vi "HFRR ADV v11.vi"() -> ()   [LabVIEW 2025] (continued)
          frame True {
          }
        }
        n2643 = In Range and Coerce(upper limit=w3178, x=w3151, lower limit=w3177) -> (In Range?=w3169:bool)  [unwired: 1 out]
        n2644 = In Range and Coerce(upper limit=w3175, x=w3150, lower limit=w3176) -> (In Range?=w3167:bool)  [unwired: 1 out]
        n2645 = case shown="True" w3183 {
          frame False {
            n2646 = local read "Rt 3"() -> (w3311:bool)
            n2647 = case shown="True" w3311 {
              frame False {
              }
              frame True {
                n2648 = local write "Rt 3"(FALSE ("Rt 3")) -> ()
                n2649 = local write "Json End Flg"(TRUE ("Upld AR 2")) -> ()
              }
            }
            "Rt" <- TRUE ("Rt")
            "Rt 2" <- FALSE ("Rt")
          }
          frame True {
            n2650 = local read "Rt"() -> (w3318:bool)
            n2651 = local write "Rt 2"(TRUE ("Rt 2")) -> ()
            n2652 = case shown="True" w3318 {
              frame False {
              }
              frame True {
                w3319 = TRUE ("Upld AR 2")
                n2653 = local write "Rt"(FALSE ("Rt")) -> ()
                n2654 = local write "Upld AR"(w3319) -> ()
                n2655 = local write "Json St Flg"(w3319) -> ()
              }
            }
            "Rt 3" <- TRUE ("Rt 3")
          }
        }
        n2656 = case shown="True" w3169 {
          tunnel: [FALSE ("RUN") TRUE ("RUN")] -> w3168
          tunnel: [_ 2] -> w3162
          frame False {
          }
          frame True {
          }
        }
        n2657 = case shown="True" w3167 {
          tunnel: [FALSE ("RUN") TRUE ("RUN")] -> w3166
          tunnel: [_ 3] -> w3161
          frame False {
          }
          frame True {
          }
        }
        n2658 = case shown="\"Acquire\"" w3147 {
          tunnel: w3149 -> [_ w3380]
          frame Default {
            w3379 = 0.0 ("output")
            n2659 = local write "PID-out"(w3379) -> ()
            n2660 = local write "Frequency ( Hz )"(w3379) -> ()
          }
          frame "Acquire" {
            n2661 = stacked-sequence {
              frame #0 {
                n2662 = local read "Auto Start Test"() -> (w3382:bool)
                n2663 = case shown="True" w3382 {
                  tunnel: "RUN" -> [w3403 w3406]
                  tunnel: [w3403 w3405] -> w3383
                  frame False {
                  }
                  frame True {
                    n2664 = local read "Auto Start Temp"() -> (w3404:bool)
                    n2665 = Or(x=w3406, y=w3404) -> (x .or. y?=w3405:bool)
                  }
                }
                n2666 = local read "clk"() -> (w3402:dbl)
                n2667 = local read "Save"() -> (w3398:bool)
                n2668 = Equal?(x=w3402, y=0.0) -> (x = y?=w3399:bool)
                n2669 = And(x=w3399, y=w3398) -> (x .and. y?=w3400:bool)
                n2670 = Not(x="Engage") -> (.not. x?=w3389:bool)
                n2671 = case shown="True" w3383 {
                  tunnel: [w3414 w3432] -> w3385
                  frame False {
                    w3414 = 0.0
                    n2672 = local read "Auto Start Test"() -> (w3410:bool)
                    n2673 = local write "Reinit PID"(TRUE) -> ()
                    n2674 = local write "Start Time"(TRUE ("Start Time")) -> ()
                    n2675 = property on="Stroke" class="DigNum (strict)"("Visible"=TRUE) -> ()  [unwired: 2 in, 2 out]
                    n2676 = property on="Stroke 2" class="DigNum (strict)"("Visible"=FALSE) -> ()  [unwired: 2 in, 2 out]
                    n2677 = case shown="False" w3410 {
                      frame False {
                        n2678 = property on="Heater Button" class="Bool (strict)"("DisabledEnum"=T16."Enabled" ("Disabled")) -> ()  [unwired: 2 in, 2 out]
                        n2679 = property on="Humidity" class="Bool (strict)"("DisabledEnum"=T16."Enabled" ("Disabled")) -> ()  [unwired: 2 in, 2 out]
                      }
                      frame True {
                      }
                    }
                    n2680 = case shown="False" "TestCompFlg" {
                      frame False {
                        n2681 = local read "StartFlg"() -> (w3420:bool)
                        n2682 = case shown="True" w3420 {
                          frame False {
                          }
                          frame True {
                            n2683 = flat-sequence {
                              frame #0 {
                                n2684 = local read "EVENT LOG"() -> (w3422:string)
                                n2685 = call "Event Log.vi"("Content"="Test was interrupted", "EVENT LOG"=w3422) -> ("EVENT LOG"=w3423:string)  [unwired: 8 in, 1 out]
                                n2686 = local write "EVENT LOG"(w3423) -> ()
                              }
                              frame #1 {
                                w3424 = FALSE ("StartFlg")
                                n2687 = local write "Heater Button"(w3424) -> ()
                                n2688 = local write "StartFlg"(w3424) -> ()
                                n2689 = local write "Humidity"(w3424) -> ()
                              }
                            }
                          }
                        }
                      }
                      frame True {
                      }
                    }
                    n2690 = local write "String 14"("Test will autostart once parameters reach the set value." ("String 14")) -> ()
                    n2691 = local write "Old Pid Val"(w3414) -> ()
                  }
                  frame True {
                    n2692 = property on="Stroke 2" class="DigNum (strict)"("Visible"=TRUE) -> ()  [unwired: 2 in, 2 out]
                    n2693 = property on="Stroke" class="DigNum (strict)"("Visible"=FALSE) -> ()  [unwired: 2 in, 2 out]
                    n2694 = property on="STOP 2" class="Bool (strict)"("Disabled"=u8 2) -> ()  [unwired: 2 in, 2 out]
                    n2695 = local write "String 14"(" Running....." ("String 14")) -> ()
                    n2696 = property on="Heater Button" class="Bool (strict)"("DisabledEnum"=T16."Disabled and Grayed Out" ("Disabled")) -> ()  [unwired: 2 in, 2 out]
                    n2697 = property on="Humidity" class="Bool (strict)"("DisabledEnum"=T16."Disabled and Grayed Out" ("Disabled")) -> ()  [unwired: 2 in, 2 out]
                    n2698 = local read "PID Ref"() -> (w3443:bool)
                    n2699 = case shown="True" w3443 {
                      tunnel: [w3449 w3465] -> w3442
                      frame False {
                        n2700 = local read "Old Pid Val"() -> (w3449:dbl)
                      }
                      frame True {
                        n2701 = local read "Set Hz"() -> (w3458:dbl)
                        n2702 = local read "Frequency"() -> (w3469:dbl)
                        n2703 = Add(x=w3458, y=10.0) -> (x+y=w3467:dbl)
                        n2704 = Add(x=w3458, y=-10.0 ("Offset")) -> (x+y=w3476:dbl)
                        n2705 = Add(x=w3458, y=-10.0) -> (x+y=w3468:dbl)
                        n2706 = In Range and Coerce(upper limit=w3467, x=w3469, lower limit=w3468) -> (coerced(x)=w3457:dbl)  [unwired: 1 out]
                        n2707 = Or(x="Reinit PID", y="Reinit PID") -> (x .or. y?=w3466:bool)
                        n2708 = Multiply(x=w3476, y=0.1 ("Gain")) -> (x*y=w3455:dbl)
                        n2709 = local read "Elapsed time"() -> (w3462:dbl)
                        n2710 = local read "SPEED OUT:"() -> (w3477:dbl)
                        n2711 = Add(x=w3455, y=1.5) -> (x+y=w3453:dbl)
                        n2712 = call-poly <vilib>:"PID.vi"("reinitialize? (F)"=w3466, "output range"=cluster{"output high":dbl, "output low":dbl} {"output high"=1.0, "output low"=-1.0}, "PID gains"=T13 {"proportional gain (Kc)"=0.0005, "integral time (Ti, min)"=0.001, "derivative time (Td, min)"=0.0} ("Motor PID"), "process variable"=w3457, "setpoint"=w3458) -> ("output"=w3456:dbl)  [unwired: 5 in, 1 out]
                        n2713 = Multiply(x=w3453, y=w3477) -> (x*y=w3452:dbl)
                        n2714 = Greater?(x=w3462, y=0.05) -> (0:w3461:bool)
                        n2715 = case shown="True" w3461 {
                          tunnel: w3456 -> [_ w3479]
                          tunnel: [0.0 ("output") w3479] -> w3459
                          frame False {
                          }
                          frame True {
                            n2716 = local write "Reinit PID"(FALSE ("Reinit PID")) -> ()
                          }
                        }
                        n2717 = Multiply(x=w3452, y=0.8) -> (x*y=w3451:dbl)
                        n2718 = Add(x=w3451, y=w3459) -> (x+y=w3464:dbl)
                        n2719 = flat-sequence {
                          tunnel: [w3482] -> w3465
                          tunnel: w3464 -> [w3482]
                          frame #0 {
                            n2720 = local write "PID Ref"(FALSE ("PID Ref")) -> ()
                          }
                        }
                      }
                    }
                    "Old Pid Val" <- w3442
                    n2721 = case shown="True" "Start Time" {
                      selector: "Start Time" -> [_ w3445]
                      frame False {
                      }
                      frame True {
                        n2722 = Not(x=w3445) -> (.not. x?=w3444:bool)
                        n2723 = local write "Start Time"(w3444) -> ()
                        n2724 = local read "EVENT LOG"() -> (w3446:string)
                        n2725 = call "Event Log.vi"("Content"="Test in progress", "EVENT LOG"=w3446) -> ("EVENT LOG"=w3448:string)  [unwired: 8 in, 1 out]
                        n2726 = local write "EVENT LOG"(w3448) -> ()
                      }
                    }
                    n2727 = local read "Set Hz"() -> (w3439:dbl)
                    n2728 = call <vilib>:"Uniform White Noise Waveform.vi"() -> ("signal out"=w3438:waveform(dbl))  [unwired: 10 in, 1 out]
                    n2729 = local read "Freq"() -> (w3431:dbl)
                    n2730 = Add(x=w3439, y=w3438) -> (x+y=w3437:waveform(dbl))
                    n2731 = Multiply(x=w3437, y=ext 0.1) -> (x*y=w3433:waveform(ext))
                    n2732 = Multiply(x=w3431, y=0.9) -> (x*y=w3434:dbl)
                    n2733 = Add(x=w3433, y=w3434) -> (x+y=w3432:waveform(ext))
                    "StartFlg" <- TRUE ("StartFlg")
                  }
                }
                n2734 = case shown="True" w3400 {
                  frame False {
                  }
                  frame True {
                    n2735 = local write "clk"(10.0 ("clk")) -> ()
                    n2736 = Get Date/Time In Seconds() -> (seconds since 1Jan1904=w3485:timestamp)
                    n2737 = To Double Precision Float(number=w3485) -> (double precision float=w3483:dbl)
                    n2738 = local write "acq timer"(w3483) -> ()
                    n2739 = local write "act save time"(w3483) -> ()
                  }
                }
                n2740 = call "Elapsed Time"("Time Target (s)"="Countdown", "Reset"=w3389) -> ("Elapsed Time (s)"=w3394:dbl, "Time has Elapsed"=w3392:bool)  [unwired: 10 in, 6 out]
                "Countdown 2" <- w3394
                n2741 = Subtract(x=w3394, y=2.0) -> (x-y=w3397:dbl)
                n2742 = Less?(x=w3397, y="Countdown") -> (x < y?=w3395:bool)
                n2743 = And(x=w3395, y=w3392) -> (x .and. y?=w3391:bool)
                n2744 = case shown="True" w3391 {
                  frame False {
                  }
                  frame True {
                    (unwired) dbl[] [] ("History Data")
                    n2745 = local write "Engage"(FALSE ("Engage")) -> ()
                    n2746 = local write "RUN"(TRUE ("RUN")) -> ()
                    n2747 = local read "Humidity ( %RH )"() -> (→"Rh Before":dbl)
                  }
                }
                n2748 = local read "Test \nStatus"() -> (w3387:bool)
                n2749 = Select(t=w3385, s=w3387, f=0.0) -> (s? t:f=w3386:dbl)
                n2750 = local write "Frequency ( Hz )"(w3386) -> ()
                n2751 = local write "Freq"(w3386) -> ()
              }
              frame #1 {
                w3508 = 1000000.0 ("x")
                # "Elapsed time\ncof\nstroke\nAir temp\nTemp\nHumidity"
                # "acq timer\n\nact save time"
                # "convert to microseconds"
                n2752 = local read "COUNT"() -> (w3491:i32)
                n2753 = local read "Rate"() -> (w3504:dbl)
                n2754 = Divide(x=w3508, y=w3504) -> (x/y=w3509:dbl)
                n2755 = Greater Or Equal?(x=w3491, y=250) -> (x >= y?=w3490:bool)
                n2756 = Get Date/Time In Seconds() -> (seconds since 1Jan1904=w3511:timestamp)
                n2757 = case shown="True" w3490 {
                  frame False {
                    n2758 = local read "COUNT"() -> (w3512:i32)
                    n2759 = Increment(x=w3512) -> (x+1=w3513:i32)
                    n2760 = local write "COUNT"(w3513) -> ()
                  }
                  frame True {
                    n2761 = local write "COUNT"(0 ("COUNT")) -> ()
                  }
                }
                n2762 = local read "Samplingtime 2"() -> (w3489:dbl)
                n2763 = local read "act save time"() -> (w3506:dbl)
                n2764 = Divide(x=w3509, y=w3508) -> (x/y=w3507:dbl)
                n2765 = To Double Precision Float(number=w3511) -> (double precision float=w3500:dbl)
                n2766 = Add(x=w3506, y=w3489) -> (x+y=w3505:dbl)
                n2767 = local read "acq timer"() -> (w3510:dbl)
                n2768 = local read "COUNT"() -> (w3493:i32)
                n2769 = Greater Or Equal?(x=w3500, y=w3505) -> (x >= y?=w3488:bool)
                n2770 = Multiply(x=w3507, y=w3493) -> (x*y=w3499:dbl)
                n2771 = Subtract(x=w3500, y=w3510) -> (x-y=w3502:dbl)
                n2772 = local read "Save"() -> (w3503:bool)
                n2773 = Add(x=w3502, y=w3499) -> (x+y=w3486:dbl)
                "Elapsed time 3" <- w3486
                n2774 = And(x=w3488, y=w3503) -> (x .and. y?=w3501:bool)
                n2775 = Divide(x=w3486, y=60.0) -> (x/y=w3497:dbl)
                n2776 = local read "Test \nStatus"() -> (w3487:bool)
                n2777 = local read "clk"() -> (w3494:dbl)
                n2778 = Equal?(x=w3494, y=10.0) -> (x = y?=w3496:bool)
                n2779 = case shown="True" w3501 {
                  tunnel: w3500 -> [_ w3615]
                  tunnel: [FALSE ("Boolean 2") TRUE ("Boolean 2")] -> _
                  frame False {
                  }
                  frame True {
                    w3562 = ";" ("Substring")
                    # "Pid out/\nFreq response value"
                    n2780 = local write "act save time"(w3615) -> ()
                    n2781 = local read "FILE"() -> (w3556:string)
                    n2782 = call "file check.vi"("file name in"=w3556) -> ("error out"=w3559:errorcluster, "file name out"=w3554:string)  [unwired: 9 in]
                    n2783 = call "FILE PATH CREATION.vi"("error in"=w3559, "FILE NAME :"=w3554) -> ("FILE OUT"=w3557:path)  [unwired: 8 in, 1 out]
                    n2784 = Concatenate Strings(w3554, ".dgf" ("Substring")) -> (w3558:string)
                    n2785 = local read "Set Strk"() -> (w3586:dbl)
                    n2786 = local read "Stroke"() -> (w3577:dbl)
                    n2787 = local read "FF 2"() -> (→"Frictional Force ( N )" →"Frictional Force ( N )":dbl)
                    n2788 = Build Path(base path=w3557, name or relative path=w3558) -> (appended path=w3553:path)
                    n2789 = Subtract(x=w3577, y=w3586) -> (x-y=w3583:dbl)
                    n2790 = local read "COF 2"() -> (w3568:dbl)
                    "cof" <- w3568
                    "Coefficient of Friction" <- w3568
                    "COF 4" <- w3568
                    "Coefficient of Friction" <- w3568
                    n2791 = Multiply(x=w3583, y=0.05) -> (x*y=w3585:dbl)
                    n2792 = local read "TEMP"() -> (w3572:dbl)
                    "Temp" <- w3572
                    "Temperature ( Deg C )" <- w3572
                    n2793 = Add(x=w3585, y=w3586) -> (x+y=w3566:dbl)
                    "Stroke Ln" <- w3566
                    "Disp" <- w3566
                    n2794 = local read "ecr"() -> (w3569:dbl)
                    "Electrical Contact Resistance ( % )" <- w3569
                    n2795 = local read "Humidity ( %RH )"() -> (w3571:dbl)
                    "Humidity ( %RH )" <- w3571
                    "Humidity ( %RH )" <- w3571
                    n2796 = local read "Frequency ( Hz )"() -> (w3579:dbl)
                    n2797 = local read "Elapsed time"() -> (w3608:dbl)
                    n2798 = disable-structure shown="Disabled" {
                      frame Disabled {
                        n2799 = local read "ecr 3"() -> ()  [unwired: 1 in]
                      }
                      frame Enabled {
                      }
                    }
                    n2800 = local read "AIR TEMP"() -> (w3576:dbl)
                    n2801 = local read "PID-out"() -> (w3582:dbl)
                    n2802 = local write "Temperature ( Deg C )"(w3572) -> ()
                    n2803 = Number To Fractional String(number=w3566, width (-)=i16 9 ("precision (6)"), precision (6)=i16 6) -> (F-format string=w3601:string)  [unwired: 1 in]
                    n2804 = Number To Fractional String(number=w3576, width (-)=i16 9 ("precision (6)"), precision (6)=i16 3) -> (F-format string=w3600:string)  [unwired: 1 in]
                    n2805 = Number To Fractional String(number=w3572, width (-)=i16 9 ("precision (6)"), precision (6)=i16 3) -> (F-format string=w3597:string)  [unwired: 1 in]
                    n2806 = Number To Fractional String(number=w3571, width (-)=i16 9 ("precision (6)"), precision (6)=i16 3) -> (F-format string=w3594:string)  [unwired: 1 in]
                    n2807 = Number To Fractional String(number=w3569, width (-)=i16 9 ("precision (6)"), precision (6)=i16 3) -> (F-format string=w3591:string)  [unwired: 1 in]
                    n2808 = Number To Fractional String(number=w3582, width (-)=i16 9 ("precision (6)"), precision (6)=i16 3) -> (F-format string=w3587:string)  [unwired: 1 in]
                    n2809 = Number To Fractional String(number=w3579, width (-)=i16 9 ("precision (6)"), precision (6)=i16 3) -> (F-format string=w3578:string)  [unwired: 1 in]
                    n2810 = Number To Fractional String(number=w3568, width (-)=i16 9 ("precision (6)"), precision (6)=i16 6) -> (F-format string=w3609:string)  [unwired: 1 in]
                    n2811 = Number To Fractional String(number=w3608, width (-)=i16 14 ("precision (6)"), precision (6)=i16 3) -> (F-format string=w3610:string)  [unwired: 1 in]
                    n2812 = Bundle("y"=1.02, w3566, "y"=0.98) -> (w3570:cluster{"y":dbl, dbl, "y":dbl})  [unwired: 1 in]
                    n2813 = Number To Fractional String(number="Ambient Humidity :", width (-)=i16 9 ("precision (6)"), precision (6)=i16 6) -> (F-format string=w3560:string)  [unwired: 1 in]
                    n2814 = local read "RUN"() -> (w3567:bool)
                    n2815 = case shown="True" w3567 {
                      tunnel: w3570 -> [_ w3620]
                      tunnel: w3566 -> [_ w3619]
                      tunnel: w3566 -> [_ w3618]
                      tunnel: w3566 -> [_ w3617]
                      frame False {
                      }
                      frame True {
                        "Stroke ( mm )" <- w3620
                        "Stroke ( mm )" <- w3620
                        "Stroke 4" <- w3619
                        "Stroke 3" <- w3618
                        "Stroke 2" <- w3617
                      }
                    }
                    n2816 = Concatenate Strings(w3610, w3562, w3609, w3562, w3601, w3562, w3600, w3562, w3597, w3562, w3594, w3562, w3591, w3562, w3587, w3562, w3578, w3562, w3560, "\r") -> (w3607:string)
                    n2817 = call <vilib>:"Write Characters To File.vi"("append to file? (new file:F)"=TRUE, "character string"=w3607, "file path (dialog if empty)"=w3553) -> ()  [unwired: 2 in, 1 out]
                    "refresh flag" <- TRUE ("refresh flag")
                  }
                }
                n2818 = case shown="True" w3487 {
                  tunnel: w3497 -> [_ w3523]
                  tunnel: w3502 -> [_ w3533]
                  tunnel: [0.0 w3529] -> _
                  tunnel: w3496 -> [_ w3528]
                  tunnel: [0.0 w3527] -> _
                  tunnel: w3486 -> [_ w3527]
                  tunnel: w3500 -> [w3516 _]
                  frame False {
                    n2819 = local write "acq timer"(w3516) -> ()
                    n2820 = local write "Test Duration Status"(0.0 ("Test Duration Status")) -> ()
                  }
                  frame True {
                    n2821 = local read "Set Hz"() -> (w3530:dbl)
                    n2822 = local write "Elapsed time"(w3523) -> ()
                    n2823 = local read "test time"() -> (w3522:dbl)
                    n2824 = Multiply(x=w3533, y=w3530) -> (x*y=w3532:dbl)
                    n2825 = case shown="False" w3528 {
                      tunnel: w3532 -> [w3534 _]
                      tunnel: [w3534 1.0] -> w3529
                      frame False {
                        n2826 = local write "Cycles elapsed"(w3534) -> ()
                      }
                      frame True {
                      }
                    }
                    n2827 = Greater?(x=w3523, y=w3522) -> (0:w3531:bool)
                    n2828 = Subtract(x=w3522, y=w3523) -> (x-y=w3521:dbl)
                    "time" <- w3521
                    n2829 = Multiply(x=w3521, y=60.0) -> (x*y=w3520:dbl)
                    n2830 = local write "Time Remaining"(w3520) -> ()
                    n2831 = local write "Remaining Time"(w3520) -> ()
                    n2832 = case shown="True" w3531 {
                      frame False {
                      }
                      frame True {
                        w3536 = T16."Enabled" ("Disabled")
                        w3540 = "" ("FILE")
                        w3541 = TRUE ("Visible")
                        n2833 = local write "Humidity"(FALSE ("Humidity")) -> ()
                        n2834 = local write "RUN"(FALSE ("OK Button 2")) -> ()
                        n2835 = local write "Heater Button"(FALSE ("Heater Button")) -> ()
                        n2836 = local write "Auto Start Test"(FALSE ("Auto Start Test")) -> ()
                        n2837 = local write "TestCompFlg"(TRUE ("StpFlg")) -> ()
                        n2838 = local read "Humidity ( %RH )"() -> (→"Rh After":dbl)
                        n2839 = property on="STOP 2" class="Bool (strict)"("Disabled"=u8 0) -> ()  [unwired: 2 in, 2 out]
                        n2840 = local read "EVENT LOG"() -> (w3546:string)
                        n2841 = call "Event Log.vi"("Content"="Test Completed", "EVENT LOG"=w3546) -> ("EVENT LOG"=w3545:string)  [unwired: 8 in, 1 out]
                        n2842 = property on="RUN" class="Bool (strict)"("Visible"=w3541) -> ()  [unwired: 2 in, 2 out]
                        n2843 = property on="Auto Start Test" class="Bool (strict)"("Visible"=w3541) -> ()  [unwired: 2 in, 2 out]
                        n2844 = local write "Batch Ref Num :"(w3540) -> ()
                        n2845 = local write "FILE"(w3540) -> ()
                        n2846 = local write "EVENT LOG"(w3545) -> ()
                        n2847 = local write "TEST FILE NAM,E SAVED"(FALSE ("TEST FILE NAM,E SAVED")) -> ()
                        n2848 = local write "Fuel Discription :"(w3540) -> ()
                        n2849 = local write "Remarks :"(w3540) -> ()
                        n2850 = local write "Main Dashboard Buttons"(T1."Imaging" ("Main Dashboard Buttons")) -> ()
                        n2851 = local write "Main Tab"(T2."Adv Scar" ("Main Tab")) -> ()
                        n2852 = property on="FRICVALZ 2" class="Bool (strict)"("DisabledEnum"=w3536) -> ()  [unwired: 2 in, 2 out]
                        n2853 = property on="FRICVALZ 3" class="Bool (strict)"("DisabledEnum"=w3536) -> ()  [unwired: 2 in, 2 out]
                        n2854 = property on="FRICVALZ 4" class="Bool (strict)"("DisabledEnum"=w3536) -> ()  [unwired: 2 in, 2 out]
                      }
                    }
                    n2855 = Divide(x=w3523, y=w3522) -> (x/y=w3526:dbl)
                    n2856 = Multiply(x=w3526, y=100.0) -> (x*y=w3524:dbl)
                    n2857 = local write "Test Duration Status"(w3524) -> ()
                  }
                }
              }
              frame #2 {
                n2858 = case shown="True" "Heater Button" {
                  tunnel: [0.0 ("output") w3644] -> w3621
                  frame False {
                    w3624 = TRUE ("tmpchk")
                    n2859 = local read "TEMP"() -> (w3625:dbl)
                    n2860 = local write "Temp ini"(w3625) -> ()
                    n2861 = local write "Reset 4"(w3624) -> ()
                    n2862 = local write "tmpchk"(w3624) -> ()
                    n2863 = local write "reinit"(TRUE ("reinit")) -> ()
                    n2864 = local write "manual temp log"(TRUE ("manual temp log")) -> ()
                  }
                  frame True {
                    # "Logic to turn off\nthe heater when \ntemp is not rising.\nTime - 60 sec\nDelta t- 5°c"
                    n2865 = local read "Temp ini"() -> (w3632:dbl)
                    n2866 = local read "Auto Start Test"() -> (w3628:bool)
                    n2867 = Less?(x=w3632, y=53.0) -> (x < y?=w3630:bool)
                    n2868 = case shown="False" w3628 {
                      frame False {
                        n2869 = local read "Set Temp"() -> (w3655:dbl)
                        n2870 = local read "TEMP"() -> (w3654:dbl)
                        n2871 = Subtract(x=w3655, y=w3654) -> (x-y=w3653:dbl)
                        n2872 = Absolute Value(x=w3653) -> (abs(x)=w3652:dbl)
                        n2873 = Less?(x=w3652, y=0.5) -> (x < y?=w3650:bool)
                        n2874 = case shown="True" w3650 {
                          tunnel: "manual temp log" -> [_ w3656]
                          frame False {
                          }
                          frame True {
                            n2875 = case shown="True" w3656 {
                              selector: w3656 -> [_ w3657]
                              frame False {
                              }
                              frame True {
                                # "#Event log"
                                n2876 = Not(x=w3657) -> (.not. x?=w3658:bool)
                                n2877 = local write "manual temp log"(w3658) -> ()
                                n2878 = local read "EVENT LOG"() -> (w3661:string)
                                n2879 = call "Event Log.vi"("Content"="Target Temperature reached", "EVENT LOG"=w3661) -> ("EVENT LOG"=w3660:string)  [unwired: 8 in, 1 out]
                                n2880 = local write "EVENT LOG"(w3660) -> ()
                              }
                            }
                          }
                        }
                      }
                      frame True {
                        n2881 = local write "manual temp log"(TRUE ("manual temp log")) -> ()
                      }
                    }
                    n2882 = And(x="tmpchk", y=w3630) -> (x .and. y?=w3633:bool)
                    n2883 = case shown="True" w3633 {
                      frame False {
                      }
                      frame True {
                        n2884 = call "Elapsed Time8"("Time Target (s)"=300.0, "Reset"="Reset 4") -> ("Time has Elapsed"=w3663:bool)  [unwired: 10 in, 7 out]
                        n2885 = flat-sequence {
                          tunnel: w3663 -> [_]
                          frame #0 {
                            n2886 = local write "Reset 4"(FALSE ("Reset 4")) -> ()
                          }
                        }
                        n2887 = case shown="True" w3663 {
                          frame False {
                          }
                          frame True {
                            n2888 = local read "Temp ini"() -> (w3670:dbl)
                            n2889 = Add(x=w3670, y=5.0) -> (x+y=w3668:dbl)
                            n2890 = local read "TEMP"() -> (w3671:dbl)
                            n2891 = Greater?(x=w3671, y=w3668) -> (0:w3669:bool)
                            n2892 = case shown="False" w3669 {
                              frame False {
                                n2893 = local write "Heater Button"(FALSE ("Heater Button")) -> ()
                              }
                              frame True {
                                n2894 = local write "tmpchk"(FALSE ("tmpchk")) -> ()
                              }
                            }
                          }
                        }
                      }
                    }
                    n2895 = local read "Set Temp"() -> (w3641:dbl)
                    n2896 = local read "TEMP"() -> (w3635:dbl)
                    n2897 = call-poly <vilib>:"PID.vi"("reinitialize? (F)"="reinit", "output range"="output range", "dt (s)"=-1.0, "PID gains"="Temp PID gains", "process variable"=w3635, "setpoint"=w3641) -> ("output"=w3638:dbl)  [unwired: 4 in, 1 out]
                    n2898 = Subtract(x=w3641, y=w3635) -> (x-y=w3643:dbl)
                    n2899 = Add(x=w3641, y=0.5) -> (x+y=w3639:dbl)
                    n2900 = Greater Or Equal?(x=w3635, y=w3639) -> ()  [unwired: 1 out]
                    n2901 = Select(t=0.0, s=FALSE, f=w3638) -> (s? t:f=w3637:dbl)
                    "PID output" <- w3637
                    n2902 = flat-sequence {
                      tunnel: w3637 -> [w3674]
                      tunnel: [w3674] -> w3644
                      frame #0 {
                        n2903 = local write "reinit"(FALSE ("reinit")) -> ()
                      }
                    }
                    n2904 = Bundle(w3643, "output"=w3637, "TEMP"=w3635) -> (→"gTEMP 3":cluster{dbl, "output":dbl, "TEMP":dbl})  [unwired: 1 in]
                  }
                }
                "PID-out" <- w3621
              }
              frame #3 {
                n2905 = local read "TEMP"() -> (w3676:dbl)
                n2906 = Greater Or Equal?(x=w3676, y="Set Temp 2") -> (x >= y?=w3681:bool)
                n2907 = case shown="True" w3681 {
                  tunnel: [FALSE TRUE] -> w3679
                  frame False {
                  }
                  frame True {
                  }
                }
                "Status 13" <- w3679
                n2908 = And(x=w3679, y="trip1 8") -> (x .and. y?=w3678:bool)
                n2909 = case shown="True" w3678 {
                  frame False {
                    n2910 = local write "Heater Trip Temp"(TRUE ("Heater Trip Temp")) -> ()
                  }
                  frame True {
                    w3684 = FALSE ("OK Button 2")
                    n2911 = case shown="True" "Heater Trip Temp" {
                      selector: "Heater Trip Temp" -> [_ w3686]
                      frame False {
                      }
                      frame True {
                        n2912 = Not(x=w3686) -> (.not. x?=w3685:bool)
                        n2913 = local read "EVENT LOG"() -> (w3689:string)
                        n2914 = local write "Heater Trip Temp"(w3685) -> ()
                        n2915 = call "Event Log.vi"("Content"="Heater Trip", "EVENT LOG"=w3689) -> ("EVENT LOG"=w3688:string)  [unwired: 8 in, 1 out]
                        n2916 = local write "EVENT LOG"(w3688) -> ()
                      }
                    }
                    n2917 = local write "RUN"(w3684) -> ()
                    n2918 = property on="Auto Start Test" class="Bool (strict)"("Value"=w3684) -> ()  [unwired: 2 in, 2 out]
                    n2919 = local write "Heater Button"(w3684) -> ()
                  }
                }
              }
            }
            n2920 = case shown="False" w3380 {
              frame False {
                n2921 = disable-structure shown="Enabled" {
                  frame Enabled {
                    n2922 = stacked-sequence {
                      frame #0 {
                        n2923 = local write "RUN"(FALSE ("OK Button 2")) -> ()
                      }
                      frame #1 {
                      }
                    }
                  }
                  frame Disabled {
                  }
                }
              }
              frame True {
              }
            }
          }
        }
        n2924 = local read "airtempflg"() -> (w3172:bool)
        n2925 = Or(x=w3172, y=w3170) -> (x .or. y?=w3173:bool)
        n2926 = Insert Into Array(array=string[] ["Air Temperature has reached set value,", "Humidity has reached set value,", "Sample Temperaturehas reached set value,", ""], index=0, new element="") -> (w3158:string[])
        n2927 = Build Array(w3163, w3162, w3161) -> (w3159:i32[])
        n2928 = disable-structure shown="Disabled" {
          disable-tunnel: w3173 -> [w3250 _]
          disable-tunnel: w3168 -> [w3249 _]
          disable-tunnel: w3166 -> [w3248 _]
          frame Disabled {
            n2929 = Compound Arithmetic op=AND(w3250, w3249, w3248) -> ()  [unwired: 1 out]
            n2930 = case shown="True" {
              selector: _ -> [_ _]
              frame False {
              }
              frame True {
                w3251 = FALSE ("autostrtflg")
                n2931 = local write "RUN"(TRUE ("RUN")) -> ()
                n2932 = local write "autostrtflg"(w3251) -> ()
                n2933 = local write "autostart"(w3251) -> ()
                n2934 = local write "String 14"(" Running....." ("String 14")) -> ()
              }
            }
          }
          frame Enabled {
          }
        }
        n2935 = for {
          tunnel: w3159 -> [w3301] mode=indexing
          tunnel: w3158 -> [w3300]
          shift-right: [w3297] -> w3157
          shift-left: "" -> [w3299]
          n2936 = Index Array(array=w3300, index=w3301) -> (element=w3298:string)
          n2937 = Concatenate Strings(w3298, w3299) -> (w3297:string)
        }
        n2938 = local write "autostart 2"(w3157) -> ()
        n2939 = local read "Reset Graph"() -> (w3146:bool)
        n2940 = case shown="True" w3146 {
          selector: w3146 -> [_ w3200]
          frame False {
          }
          frame True {
            w3214 = 0.0 ("X Scale.Range:Maximum")
            n2941 = Not(x=w3200) -> (.not. x?=w3199:bool)
            n2942 = local write "Reset Graph"(w3199) -> ()
            n2943 = property on="Electrical Contact Resistance ( % )" class="WFChart (strict)"("XScale.Maximum"=600.0 ("X Scale.Range:Maximum"), "XScale.Minimum"=0.0 ("X Scale.Range:Minimum"), "YScale.Maximum"=100.0 ("Y Scale.Range:Maximum"), "YScale.Minimum"=0.0 ("Y Scale.Range:Minimum")) -> ()  [unwired: 2 in, 2 out]
            n2944 = property on="Frictional Force ( N )" class="WFChart (strict)"("XScale.Maximum"=600.0 ("X Scale.Range:Maximum"), "XScale.Minimum"=0.0 ("X Scale.Range:Minimum"), "YScale.Maximum"=100.0 ("Y Scale.Range:Maximum"), "YScale.Minimum"=0.0 ("Y Scale.Range:Minimum")) -> ()  [unwired: 2 in, 2 out]
            n2945 = property on="Temperature ( Deg C )" class="WFChart (strict)"("XScale.Maximum"=600.0 ("X Scale.Range:Maximum"), "XScale.Minimum"=0.0 ("X Scale.Range:Minimum"), "YScale.Maximum"=100.0 ("Y Scale.Range:Maximum"), "YScale.Minimum"=0.0 ("Y Scale.Range:Minimum")) -> ()  [unwired: 2 in, 2 out]
            n2946 = property on="Humidity ( %RH )" class="WFChart (strict)"("XScale.Maximum"=600.0 ("X Scale.Range:Maximum"), "XScale.Minimum"=0.0 ("X Scale.Range:Minimum"), "YScale.Maximum"=100.0 ("Y Scale.Range:Maximum"), "YScale.Minimum"=0.0 ("Y Scale.Range:Minimum")) -> ()  [unwired: 2 in, 2 out]
            n2947 = property on="Stroke ( mm )" class="WFChart (strict)"("XScale.Maximum"=600.0 ("X Scale.Range:Maximum"), "XScale.Minimum"=0.0 ("X Scale.Range:Minimum"), "YScale.Maximum"=100.0 ("Y Scale.Range:Maximum"), "YScale.Minimum"=0.0 ("Y Scale.Range:Minimum")) -> ()  [unwired: 2 in, 2 out]
            n2948 = property on="Coefficient of Friction" class="WFChart (strict)"("XScale.Maximum"=600.0 ("X Scale.Range:Maximum"), "XScale.Minimum"=0.0 ("X Scale.Range:Minimum"), "YScale.Maximum"=100.0 ("Y Scale.Range:Maximum"), "YScale.Minimum"=0.0 ("Y Scale.Range:Minimum")) -> ()  [unwired: 2 in, 2 out]
            n2949 = property on="Electrical Contact Resistance ( % )" class="WFChart (strict)"("XScale.Minimum"=0.0 ("X Scale.Range:Minimum"), "XScale.Maximum"=600.0 ("X Scale.Range:Maximum"), "YScale.Minimum"=0.0 ("Y Scale.Range:Minimum"), "YScale.Maximum"=100.0 ("Y Scale.Range:Maximum")) -> ()  [unwired: 2 in, 2 out]
            n2950 = property on="Temperature ( Deg C )" class="WFChart (strict)"("XScale.Minimum"=0.0 ("X Scale.Range:Minimum"), "XScale.Maximum"=600.0 ("X Scale.Range:Maximum"), "YScale.Minimum"=0.0 ("Y Scale.Range:Minimum"), "YScale.Maximum"=100.0 ("Y Scale.Range:Maximum")) -> ()  [unwired: 2 in, 2 out]
            n2951 = property on="Coefficient of Friction" class="WFChart (strict)"("XScale.Minimum"=0.0 ("X Scale.Range:Minimum"), "XScale.Maximum"=600.0 ("X Scale.Range:Maximum"), "YScale.Maximum"=1.0 ("X Scale.Range:Minimum"), "YScale.Minimum"=0.0 ("X Scale.Range:Minimum")) -> ()  [unwired: 2 in, 2 out]
            n2952 = property on="Frictional Force ( N )" class="WFChart (strict)"("XScale.Maximum"=600.0 ("X Scale.Range:Maximum"), "XScale.Minimum"=w3214, "YScale.Maximum"=10.0 ("Y Scale.Range:Maximum"), "YScale.Minimum"=w3214) -> ()  [unwired: 2 in, 2 out]
            n2953 = property on="Stroke ( mm )" class="WFChart (strict)"("XScale.Maximum"=600.0 ("X Scale.Range:Maximum"), "XScale.Minimum"=0.0 ("X Scale.Range:Minimum"), "YScale.Maximum"=100.0 ("Y Scale.Range:Maximum"), "YScale.Minimum"=0.0 ("Y Scale.Range:Minimum")) -> ()  [unwired: 2 in, 2 out]
            n2954 = property on="Humidity ( %RH )" class="WFChart (strict)"("XScale.Maximum"=600.0 ("X Scale.Range:Maximum"), "XScale.Minimum"=0.0 ("X Scale.Range:Minimum"), "YScale.Maximum"=100.0 ("Y Scale.Range:Maximum"), "YScale.Minimum"=0.0 ("Y Scale.Range:Minimum")) -> ()  [unwired: 2 in, 2 out]
          }
        }
      }
      frame "Compare Files" {
        # "Elapsed time\ncof\nstroke\nAir temp\nTemp\nHumidity"
        n2955 = case shown="True" "RSTV1 2" {
          frame False {
          }
          frame True {
            n2956 = property on="Humidity ( %RH )" class="XYGraph (strict)"("Y Scale.Display Format:Precision"=u8 0 ("Y Scale.Format & Precision:Precision")) -> ()  [unwired: 2 in, 2 out]
            n2957 = property on="Humidity ( %RH )" class="XYGraph (strict)"("X Scale.Range:Minimum"=0.0, "X Scale.Range:Maximum"=75.0, "Y Scale.Range:Minimum"=48.0, "Y Scale.Range:Maximum"=58.0) -> ()  [unwired: 2 in, 2 out]
          }
        }
        n2958 = case shown="True" "RST CP 2" {
          frame False {
          }
          frame True {
            n2959 = property on="XY Graph 13" class="XYGraph (strict)"("Y Scale.Display Format:Precision"=u8 0 ("Y Scale.Format & Precision:Precision")) -> ()  [unwired: 2 in, 2 out]
            n2960 = property on="XY Graph 13" class="XYGraph (strict)"("X Scale.Range:Minimum"=0.0, "X Scale.Range:Maximum"=75.0, "Y Scale.Range:Minimum"=0.0, "Y Scale.Range:Maximum"=100.0) -> ()  [unwired: 2 in, 2 out]
          }
        }
        n2961 = case shown="True" "RST CP" {
          frame False {
          }
          frame True {
            n2962 = property on="Sample Temperature ( °C )" class="XYGraph (strict)"("Y Scale.Display Format:Precision"=u8 2 ("Y Scale.Format & Precision:Precision")) -> ()  [unwired: 2 in, 2 out]
            n2963 = property on="Sample Temperature ( °C )" class="XYGraph (strict)"("X Scale.Range:Minimum"=0.0, "X Scale.Range:Maximum"=75.0, "Y Scale.Range:Minimum"=58.0, "Y Scale.Range:Maximum"=62.0) -> ()  [unwired: 2 in, 2 out]
          }
        }
        n2964 = case shown="True" "RSTV1 3" {
          frame False {
          }
          frame True {
            n2965 = property on="Air Temperature  ( °C )" class="XYGraph (strict)"("Y Scale.Display Format:Precision"=u8 2 ("Y Scale.Format & Precision:Precision")) -> ()  [unwired: 2 in, 2 out]
            n2966 = property on="Air Temperature  ( °C )" class="XYGraph (strict)"("X Scale.Range:Minimum"=0.0 ("Y Scale.Range:Minimum"), "X Scale.Range:Maximum"=75.0 ("Y Scale.Range:Maximum"), "Y Scale.Range:Minimum"=20.0 ("X Scale.Range:Minimum"), "Y Scale.Range:Maximum"=26.0 ("X Scale.Range:Maximum")) -> ()  [unwired: 2 in, 2 out]
          }
        }
        n2967 = case shown="True" "RSTV1 4" {
          frame False {
          }
          frame True {
            n2968 = property on="Stroke ( mm )" class="XYGraph (strict)"("Y Scale.Display Format:Precision"=u8 2 ("Y Scale.Format & Precision:Precision")) -> ()  [unwired: 2 in, 2 out]
            n2969 = property on="Stroke ( mm )" class="XYGraph (strict)"("X Scale.Range:Minimum"=0.0 ("Y Scale.Range:Maximum"), "X Scale.Range:Maximum"=75.0 ("X Scale.Range:Minimum"), "Y Scale.Range:Minimum"=0.98, "Y Scale.Range:Maximum"=1.02) -> ()  [unwired: 2 in, 2 out]
          }
        }
        n2970 = case shown="True" "rstv2" {
          frame False {
          }
          frame True {
            n2971 = property on="Coefficient Of Friction" class="XYGraph (strict)"("Y Scale.Display Format:Precision"=u8 3 ("Y Scale.Format & Precision:Precision")) -> ()  [unwired: 2 in, 2 out]
            n2972 = property on="Coefficient Of Friction" class="XYGraph (strict)"("X Scale.Range:Minimum"=0.0 ("Y Scale.Range:Maximum"), "X Scale.Range:Maximum"=75.0, "Y Scale.Range:Minimum"=0.0, "Y Scale.Range:Maximum"=1.0 ("X Scale.Range:Minimum")) -> ()  [unwired: 2 in, 2 out]
          }
        }
        n2973 = case shown="True" "RST CP 3" {
          frame False {
          }
          frame True {
            n2974 = property on="Air Temp ( °C ) vs Humidity ( % RH )" class="XYGraph (strict)"("X Scale.Range:Minimum"=18.0, "X Scale.Range:Maximum"=28.0 ("X Scale.Range:Minimum"), "Y Scale.Range:Minimum"=30.0 ("X Scale.Range:Minimum"), "Y Scale.Range:Maximum"=70.0 ("X Scale.Range:Minimum")) -> ()  [unwired: 2 in, 2 out]
          }
        }
        n2975 = case shown="True" "OPEN 1" {
          frame False {
          }
          frame True {
            (unwired) 0  # existing file
            w3965 = "Choose a datalog file to open"  # prompt
            n2976 = local write "OPEN 1"(FALSE ("OPEN 1")) -> ()
            n2977 = String To Path(string="C:\\LAB-IQ\\Data\\") -> (path=w3950:path)
            n2978 = File Dialog(6:"*.dgf" ("pattern"), 7:w3965, 11:w3950) -> (0:w3948:errorcluster, 3:w3956:path)  [unwired: 4 in, 2 out]
            n2979 = Unbundle(w3948) -> ()  [unwired: 3 out]
            n2980 = Strip Path(path=w3956) -> (name=w3955:string)  [unwired: 1 out]
            n2981 = Path To String(path=w3956) -> (string=w3951:string)
            "string1" <- w3951
            n2982 = Match Pattern(string=w3955, regular expression=".dgf") -> (before substring=→"String Control":string)  [unwired: 1 in, 3 out]
            n2983 = Match Pattern(string=w3951, regular expression=".dgf" ("substring (\"\")")) -> (before substring=w3961:string)  [unwired: 1 in, 3 out]
            n2984 = Concatenate Strings(w3961, ".duf" ("Substring")) -> (w3957:string)
            n2985 = String To Path(string=w3957) -> (path=w3962:path)
            n2986 = call <vilib>:"Read Characters From File.vi"("file path (dialog if empty)"=w3962, "start of read offset (chars.:0)"=60 ("start of read offset (chars.: 0)")) -> ("character string"=→"String Control 2":string)  [unwired: 4 in, 3 out]
          }
        }
        n2987 = case shown="True" "OPEN 2" {
          frame False {
          }
          frame True {
            (unwired) 0  # existing file
            w3983 = "Choose a datalog file to open"  # prompt
            n2988 = local write "OPEN 2"(FALSE ("OPEN 1")) -> ()
            n2989 = String To Path(string="C:\\LAB-IQ\\Data\\") -> (path=w3968:path)
            n2990 = File Dialog(6:"*.dgf" ("pattern"), 7:w3983, 11:w3968) -> (0:w3966:errorcluster, 3:w3974:path)  [unwired: 4 in, 2 out]
            n2991 = Unbundle(w3966) -> ()  [unwired: 3 out]
            n2992 = Strip Path(path=w3974) -> (name=w3972:string)  [unwired: 1 out]
            n2993 = Path To String(path=w3974) -> (string=w3969:string)
            "string1 2" <- w3969
            n2994 = Match Pattern(string=w3972, regular expression=".dgf") -> (before substring=→"String Control 3":string)  [unwired: 1 in, 3 out]
            n2995 = Match Pattern(string=w3969, regular expression=".dgf" ("substring (\"\")")) -> (before substring=w3980:string)  [unwired: 1 in, 3 out]
            n2996 = Concatenate Strings(w3980, ".duf" ("Substring")) -> (w3977:string)
            n2997 = String To Path(string=w3977) -> (path=w3975:path)
            n2998 = call <vilib>:"Read Characters From File.vi"("file path (dialog if empty)"=w3975, "start of read offset (chars.:0)"=60 ("start of read offset (chars.: 0)")) -> ("character string"=→"String Control 4":string)  [unwired: 4 in, 3 out]
          }
        }
        n2999 = case shown="True" "OPEN 3" {
          frame False {
          }
          frame True {
            (unwired) 0  # existing file
            w4001 = "Choose a datalog file to open"  # prompt
            n3000 = local write "OPEN 3"(FALSE ("OPEN 1")) -> ()
            n3001 = String To Path(string="C:\\LAB-IQ\\Data\\") -> (path=w3986:path)
            n3002 = File Dialog(6:"*.dgf" ("pattern"), 7:w4001, 11:w3986) -> (0:w3984:errorcluster, 3:w3992:path)  [unwired: 4 in, 2 out]
            n3003 = Unbundle(w3984) -> ()  [unwired: 3 out]
            n3004 = Strip Path(path=w3992) -> (name=w3990:string)  [unwired: 1 out]
            n3005 = Path To String(path=w3992) -> (string=w3987:string)
            "string1 3" <- w3987
            n3006 = Match Pattern(string=w3990, regular expression=".dgf") -> (before substring=→"String Control 5":string)  [unwired: 1 in, 3 out]
            n3007 = Match Pattern(string=w3987, regular expression=".dgf" ("substring (\"\")")) -> (before substring=w3997:string)  [unwired: 1 in, 3 out]
            n3008 = Concatenate Strings(w3997, ".duf" ("Substring")) -> (w3994:string)
            n3009 = String To Path(string=w3994) -> (path=w3998:path)
            n3010 = call <vilib>:"Read Characters From File.vi"("file path (dialog if empty)"=w3998, "start of read offset (chars.:0)"=60 ("start of read offset (chars.: 0)")) -> ("character string"=→"String Control 6":string)  [unwired: 4 in, 3 out]
          }
        }
        n3011 = case shown="True" "OPEN 4" {
          frame False {
          }
          frame True {
            (unwired) 0  # existing file
            w4019 = "Choose a datalog file to open"  # prompt
            n3012 = local write "OPEN 4"(FALSE ("OPEN 1")) -> ()
            n3013 = String To Path(string="C:\\LAB-IQ\\Data\\") -> (path=w4004:path)
            n3014 = File Dialog(6:"*.dgf" ("pattern"), 7:w4019, 11:w4004) -> (0:w4002:errorcluster, 3:w4010:path)  [unwired: 4 in, 2 out]
            n3015 = Unbundle(w4002) -> ()  [unwired: 3 out]
            n3016 = Strip Path(path=w4010) -> (name=w4008:string)  [unwired: 1 out]
            n3017 = Path To String(path=w4010) -> (string=w4005:string)
            "string1 4" <- w4005
            n3018 = Match Pattern(string=w4008, regular expression=".dgf") -> (before substring=→"String Control 7":string)  [unwired: 1 in, 3 out]
            n3019 = Match Pattern(string=w4005, regular expression=".dgf" ("substring (\"\")")) -> (before substring=w4015:string)  [unwired: 1 in, 3 out]
            n3020 = Concatenate Strings(w4015, ".duf" ("Substring")) -> (w4012:string)
            n3021 = String To Path(string=w4012) -> (path=w4016:path)
            n3022 = call <vilib>:"Read Characters From File.vi"("file path (dialog if empty)"=w4016, "start of read offset (chars.:0)"=60 ("start of read offset (chars.: 0)")) -> ("character string"=→"String Control 8":string)  [unwired: 4 in, 3 out]
          }
        }
      }
      frame "About" {
        # "Elapsed time\ncof\nstroke\nmean pos\nTemp\nHumidity"
        n3023 = disable-structure shown="Disabled" {
          frame Disabled {
            n3024 = case shown="True" "Export" {
              frame False {
              }
              frame True {
                w4041 = "                                      " ("string")
                w4043 = "\r"
                (unwired) i16 6 ("width (-)")
                w4120 = "\r"
                w4052 = "\r"
                n3025 = local write "Export"(FALSE ("Export")) -> ()
                n3026 = local read "String 29"() -> (w4089:string)
                n3027 = local read "String 34"() -> (w4077:string)
                n3028 = local read "String 35"() -> (w4072:string)
                n3029 = local read "String 37"() -> (w4068:string)
                n3030 = local read "String 36"() -> (w4065:string)
                n3031 = local read "String 38"() -> (w4062:string)
                n3032 = local read "String 39"() -> (w4059:string)
                n3033 = Match Pattern(string=w4089, regular expression=".dwm") -> (before substring=w4085:string)  [unwired: 1 in, 3 out]
                "before substring" <- w4085
                n3034 = local read "S 38"() -> (w4080:string)
                n3035 = local read "S 39"() -> (w4073:string)
                n3036 = local read "Temperature before test 2"() -> (w4109:dbl)
                n3037 = local read "Temperature after test 2"() -> (w4114:dbl)
                n3038 = local read "Humidity before test 2"() -> (w4095:dbl)
                n3039 = local read "Humidity after test 2"() -> (w4110:dbl)
                n3040 = local read "MWSD 2"() -> (w4106:dbl)
                n3041 = local read "WS1.4 2"() -> (w4122:dbl)
                n3042 = local read "HCF 2"() -> (w4118:dbl)
                n3043 = local read "AVP 2"() -> (w4107:dbl)
                n3044 = Concatenate Strings("1," ("string"), w4080) -> (w4079:string)
                n3045 = Concatenate Strings("2," ("string"), w4077) -> (w4076:string)
                n3046 = Concatenate Strings("3," ("string"), w4073) -> (w4075:string)
                n3047 = Concatenate Strings("4," ("string"), w4072) -> (w4071:string)
                n3048 = Concatenate Strings("5," ("string"), w4068) -> (w4069:string)
                n3049 = Concatenate Strings("6," ("string"), w4065) -> (w4066:string)
                n3050 = Concatenate Strings("7," ("string"), w4062) -> (w4063:string)
                n3051 = Concatenate Strings("8," ("string"), w4059) -> (w4060:string)
                n3052 = local read "Sample ID"() -> (w4127:string)
                n3053 = case shown="\"xlx\"" "Select File Type" {
                  tunnel: w4085 -> [w4130 w4132 w4134]
                  tunnel: [w4128 w4133 w4135] -> w4084
                  frame "xlx" {
                    n3054 = Concatenate Strings(w4130, ".xls" ("string")) -> (w4128:string)
                  }
                  frame "csv" {
                    n3055 = Concatenate Strings(w4132, ".csv" ("string")) -> (w4133:string)
                  }
                  frame "txt" {
                    n3056 = Concatenate Strings(w4134, ".txt" ("string")) -> (w4135:string)
                  }
                }
                n3057 = local read "Test Date"() -> (w4126:string)
                n3058 = local read "String 45"() -> (w4040:string)
                n3059 = local read "String 31"() -> (w4125:string)
                n3060 = local read "String 32"() -> (w4124:string)
                n3061 = local read "TITTLE"() -> (w4048:string)
                n3062 = Number To Fractional String(number=w4095, width (-)=i16 6, precision (6)=i16 2) -> (F-format string=w4094:string)  [unwired: 1 in]
                n3063 = Number To Fractional String(number=w4109, width (-)=i16 6, precision (6)=i16 2) -> (F-format string=w4115:string)  [unwired: 1 in]
                n3064 = Number To Fractional String(number=w4110, width (-)=i16 6, precision (6)=i16 2) -> (F-format string=w4108:string)  [unwired: 1 in]
                n3065 = Number To Fractional String(number=w4114, width (-)=i16 6, precision (6)=i16 2) -> (F-format string=w4113:string)  [unwired: 1 in]
                n3066 = Number To Fractional String(number=w4106, width (-)=i16 6, precision (6)=i16 2) -> (F-format string=w4104:string)  [unwired: 1 in]
                n3067 = Number To Fractional String(number=w4107, width (-)=i16 6, precision (6)=i16 2) -> (F-format string=w4105:string)  [unwired: 1 in]
                n3068 = Number To Fractional String(number=w4118, width (-)=i16 6, precision (6)=i16 2) -> (F-format string=w4119:string)  [unwired: 1 in]
                n3069 = Number To Fractional String(number=w4122, precision (6)=i16 2) -> (F-format string=w4123:string)  [unwired: 2 in]
                n3070 = local read "s.NO"() -> (w4042:string)
                n3071 = Concatenate Strings("=" ("string"), w4048) -> (w4047:string)
                n3072 = Concatenate Strings("S.No," ("string"), "                                       Parameters" ("string")) -> (w4053:string)
                n3073 = Concatenate Strings(w4120, w4079, w4094, w4120, w4076, w4115, w4120, w4075, w4108, w4120, w4071, w4113, w4120, w4069, w4104, w4120, w4066, w4105, w4120, w4063, w4119, w4120, w4060, w4123) -> (w4082:string)
                n3074 = Concatenate Strings(w4052, "," ("string"), w4040, w4042, w4041, w4124, w4127, w4041, w4125, w4126, w4052) -> (w4050:string)
                n3075 = local read "Tested by"() -> (w4056:string)
                n3076 = local read "String 33"() -> (w4057:string)
                n3077 = Concatenate Strings("," ("string"), "                                                                             " ("string")) -> (w4045:string)
                n3078 = Concatenate Strings(w4047, w4043, w4050, w4043, w4053, w4082, w4043, w4045, w4057, w4056) -> (→"export":string)
                n3079 = String To Path(string=w4084) -> (path=w4091:path)
                n3080 = local read "export"() -> (w4086:string)
                n3081 = call <vilib>:"Write Characters To File.vi"("append to file? (new file:F)"=FALSE, "character string"=w4086, "file path (dialog if empty)"=w4091) -> ()  [unwired: 2 in, 1 out]
              }
            }
          }
          frame Enabled {
          }
        }
        n3082 = case shown="True" "OK Button 17" {
          frame False {
          }
          frame True {
            (unwired) 0  # existing file
            w4344 = "Choose a datalog file to open"  # prompt
            n3083 = local write "OK Button 17"(FALSE ("OK Button 17")) -> ()
            n3084 = local read "String"() -> (w4339:string)
            n3085 = String To Path(string=w4339) -> (path=w4340:path)
            n3086 = File Dialog(6:"*.duf" ("pattern"), 7:w4344, 11:w4340) -> (0:w4331:errorcluster, 3:w4350:path)  [unwired: 4 in, 2 out]
            n3087 = Unbundle(w4331) -> ()  [unwired: 3 out]
            n3088 = Open/Create/Replace File "Open File"(file path (use dialog)=w4350) -> (refnum out=w4342:refnum<file>)  [unwired: 5 in, 2 out]
            n3089 = Strip Path(path=w4350) -> (name=w4348:string)  [unwired: 1 out]
            n3090 = Path To String(path=w4350) -> (string=w4333:string)
            n3091 = while {
              tunnel: w4342 -> [w4354]
              i -> [w4351]
              stop <- w4352 continue-if-true
              (unwired) TRUE ("line mode (F)")
              n3092 = Read from Text File "Read File"(file (use dialog)=w4354) -> (text=w4353:string)  [unwired: 3 in, 3 out]
              n3093 = local write "Numeric 16"(w4351) -> ()
              n3094 = String Length(string=w4353) -> (length=w4356:i32)
              n3095 = Greater?(x=w4356, y=1) -> (0:w4352:bool)
            }
            n3096 = local write "String 29"(w4333) -> ()
            n3097 = Search and Replace String(input string=w4333, search string=".duf", replace string=".dgf" ("replace string (\"\")")) -> (result string=→"String Indicator 4":string)  [unwired: 5 in, 3 out]
            n3098 = Match Pattern(string=w4348, regular expression=".dwm") -> (before substring=w4332:string)  [unwired: 1 in, 3 out]
            "String Indicator" <- w4332
            n3099 = Match Pattern(string=w4333, regular expression=".dwm" ("substring (\"\")")) -> (before substring=w4334:string)  [unwired: 1 in, 3 out]
            "String Indicator 3" <- w4334
            n3100 = local write "TITTLE 2"(w4332) -> ()
            n3101 = String To Path(string=w4334) -> (path=w4341:path)
            "path" <- w4341
            n3102 = call <vilib>:"Read Characters From File.vi"("file path (dialog if empty)"=w4341, "start of read offset (chars.:0)"=60 ("start of read offset (chars.: 0)")) -> ("character string"=→"String Indicator 2":string)  [unwired: 4 in, 3 out]
          }
        }
        n3103 = call <vilib>:"Query Available Printers.vi"() -> ("system configured printers"=w4033:string[])  [unwired: 9 in, 2 out]
        "System Configured Printers 2" <- w4033
        n3104 = local read "OK Button 16"() -> (w4030:bool)
        n3105 = case shown="True" "OK Button 16" {
          frame False {
          }
          frame True {
            n3106 = stacked-sequence {
              frame #0 {
                n3107 = local read "Numeric 16"() -> (w4358:i32)
                n3108 = local write "Numeric 10"(w4358) -> ()
              }
              frame #1 {
                n3109 = local read "S.NO"() -> (→"s.NO":string)
                n3110 = local read "String 29"() -> (w4362:string)
                n3111 = String To Path(string=w4362) -> (path=w4361:path)
                n3112 = Open/Create/Replace File "Open File"(file path (use dialog)=w4361) -> (refnum out=w4363:refnum<file>)  [unwired: 5 in, 2 out]
                n3113 = for {
                  N: 16 -> [_]
                  tunnel: w4363 -> [w4370]
                  i -> [w4366]
                  (unwired) TRUE ("line mode (F)")
                  n3114 = Read from Text File "Read File"(file (use dialog)=w4370) -> (text=w4364:string)  [unwired: 3 in, 3 out]
                  n3115 = Match Pattern(string=w4364, regular expression="(") -> (after substring=w4369:string)  [unwired: 1 in, 3 out]
                  n3116 = Match Pattern(string=w4369, regular expression=")") -> (before substring=w4365:string)  [unwired: 1 in, 3 out]
                  n3117 = case shown="1" w4366 {
                    tunnel: w4365 -> [w4371 w4372 _ _ w4373 w4374 w4375 w4377 w4379 w4381 w4383 w4385 w4387 w4389 _]
                    tunnel: w4364 -> [_ _ _ _ _ _ _ _ _ _ _ _ _ _ _]
                    frame 0 {
                      "TITTLE" <- w4371
                    }
                    frame 1 {
                      "Sample ID" <- w4372
                    }
                    frame 2 {
                    }
                    frame 3 {
                    }
                    frame 4 {
                      "Test Date" <- w4373
                    }
                    frame 5 {
                      "Tested by" <- w4374
                    }
                    frame 6 {
                      n3118 = Fract/Exp String To Number(string=w4375) -> (number=→"Humidity before test 2":dbl)  [unwired: 3 in, 1 out]
                    }
                    frame 7 {
                      n3119 = Fract/Exp String To Number(string=w4377) -> (number=→"Temperature before test 2":dbl)  [unwired: 3 in, 1 out]
                    }
                    frame 8 {
                      n3120 = Fract/Exp String To Number(string=w4379) -> (number=→"Humidity after test 2":dbl)  [unwired: 3 in, 1 out]
                    }
                    frame 9 {
                      n3121 = Fract/Exp String To Number(string=w4381) -> (number=→"Temperature after test 2":dbl)  [unwired: 3 in, 1 out]
                    }
                    frame 10 {
                      n3122 = Fract/Exp String To Number(string=w4383) -> (number=→"MWSD 2":dbl)  [unwired: 3 in, 1 out]
                    }
                    frame 11 {
                      n3123 = Fract/Exp String To Number(string=w4385) -> (number=→"AVP 2":dbl)  [unwired: 3 in, 1 out]
                    }
                    frame 12 {
                      n3124 = Fract/Exp String To Number(string=w4387) -> (number=→"HCF 2":dbl)  [unwired: 3 in, 1 out]
                    }
                    frame 13 {
                      n3125 = Fract/Exp String To Number(string=w4389) -> (number=→"WS1.4 2":dbl)  [unwired: 3 in, 1 out]
                    }
                    frame 14, Default {
                    }
                  }
                }
              }
              frame #2 {
              }
            }
            n3126 = local write "OK Button 16"(FALSE ("OK Button 13")) -> ()
          }
        }
        n3127 = Index Array(array=w4033, index="Select Printer 3") -> (element=w4035:string)
        "Selected Printer" <- w4035
        n3128 = case shown="True" w4030 {
          frame False {
          }
          frame True {
            n3129 = flat-sequence {
              frame #0 {
              }
              frame #1 {
                n3130 = Wait (ms)(milliseconds to wait=u32 100) -> ()  [unwired: 1 out]
              }
              frame #2 {
                n3131 = local write "OK Button 16"(FALSE ("Print 3")) -> ()
              }
            }
          }
        }
        n3132 = case shown="True" "Print" {
          tunnel: w4035 -> [_ w4327]
          frame False {
